vi "Init HTTP (SubVI).vi"(11 "Application Key":string) -> (0 "error out":errorcluster, 3 "Refnum out":T1)   [LabVIEW 2018]
uses:
  <vilib>/httpClient/ClientHandle.ctl
  <vilib>/httpClient/LabVIEWHTTPClient.lvlib
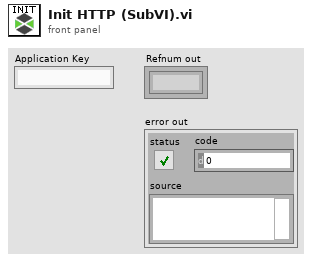
[diagram p1: front panel]
types:
  T1 = typedef "LabVIEWHTTPClient.lvlib/ClientHandle.ctl" = refnum<k1>
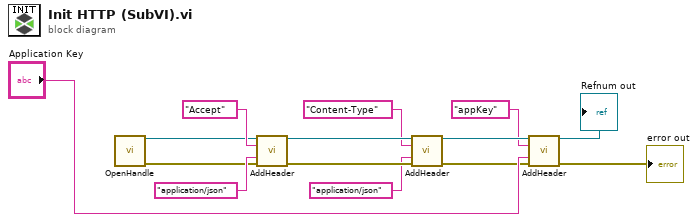
[diagram p0: block diagram]
diagram:
  n1 = call <vilib>:"OpenHandle.vi"() -> ("client handle out"=w1:T1, "error out"=w2:errorcluster)  [unwired: 14 in]
  n2 = call <vilib>:"AddHeader.vi"("client handle"=w1, "header"="Accept", "value"="application/json", "error in (no error)"=w2) -> ("client handle out"=w7:T1, "error out"=w8:errorcluster)  [unwired: 10 in]
  n3 = call <vilib>:"AddHeader.vi"("client handle"=w7, "header"="Content-Type", "value"="application/json", "error in (no error)"=w8) -> ("client handle out"=w10:T1, "error out"=w11:errorcluster)  [unwired: 10 in]
  n4 = call <vilib>:"AddHeader.vi"("client handle"=w10, "header"="appKey", "value"="Application Key", "error in (no error)"=w11) -> ("client handle out"=→"Refnum out":T1, "error out"=→"error out":errorcluster)  [unwired: 10 in]
